vi "Set DDS Bias Mv.vi"(10 "bias":i32, 11 "channel_index":u8) -> ()   [LabVIEW 2021, in "vmmso.lvlib"]
doc: "DLL_API void WINAPI SetDDSBiasMv(unsigned char channel_index, int bias);"
uses:
  vmmso.lvlib
  vmmso.dll
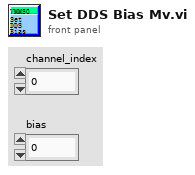
[diagram p1: front panel]
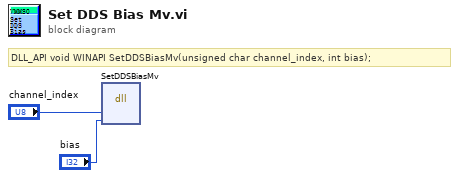
[diagram p0: block diagram]
diagram:
  # "DLL_API void WINAPI SetDDSBiasMv(unsigned char channel_index, int bias);"
  n1 = dll-call lib="D:/labviewdemo/LabviewDemo 21/vmmso/vmmso.*" fn="SetDDSBiasMv"("channel_index"="channel_index", "bias"="bias") -> ()  [unwired: 6 in, 2 out]
